vi "Deadband.vi"(10 "Deadband":dbl, 11 "Input":dbl) -> (3 "Output":dbl)   [LabVIEW 2013]
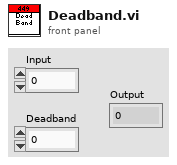
[diagram p1: front panel]
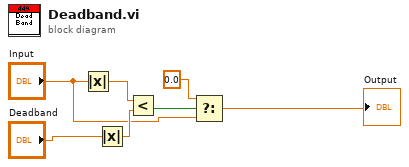
[diagram p0: block diagram]
diagram:
  n1 = Absolute Value(x="Input") -> (abs(x)=w7:dbl)
  n2 = Absolute Value(x="Deadband") -> (abs(x)=w5:dbl)
  n3 = Less?(x=w7, y=w5) -> (x < y?=w4:bool)
  n4 = Select(t=0.0, s=w4, f="Input") -> (s? t:f=→"Output":dbl)
